vi "Welcome.vi"() -> ()   [LabVIEW 2017]
uses:
  Global/Global 1.vi
  Global/Login Details.vi
  Control/WELCOM SCREEN ENUM.ctl
panel:
  out "Screen Index":i32
  in  "Check 2":bool
  in  "auto":bool
  in  "Test Print":bool
  in  "andon":bool
  in  "MANUAL":bool
  out "error out 2":errorcluster
  in  "error in (no error) 3":errorcluster
  in  "Remove":bool
  in  "Check":bool
  in  "Home":bool
  out "user name":string
  out "STOP":bool
  in  "Tab Control":enum32{"Page 1", "user mangement"}(tab)
  out "error out":errorcluster
  in  "error in (no error)":errorcluster
  in  "LOGIN":bool
  in  "RECIPE":bool
  in  "EXIT":bool
  in  "REPORT":bool
  in  "Hardware Setting":bool
  in  "Shift Setting":bool
  in  "AUTO MODE":bool
  in  "USER MANGMENT":bool
  out "datetime":string
  # "PV Clean Mobility Technologies Traceability System"
  # "USER :"
  # "Powered By - NiVision Automation Systems Pvt. Ltd."
  # "Powered By-Infinity Automation Systems Pvt Ltd. Pune"
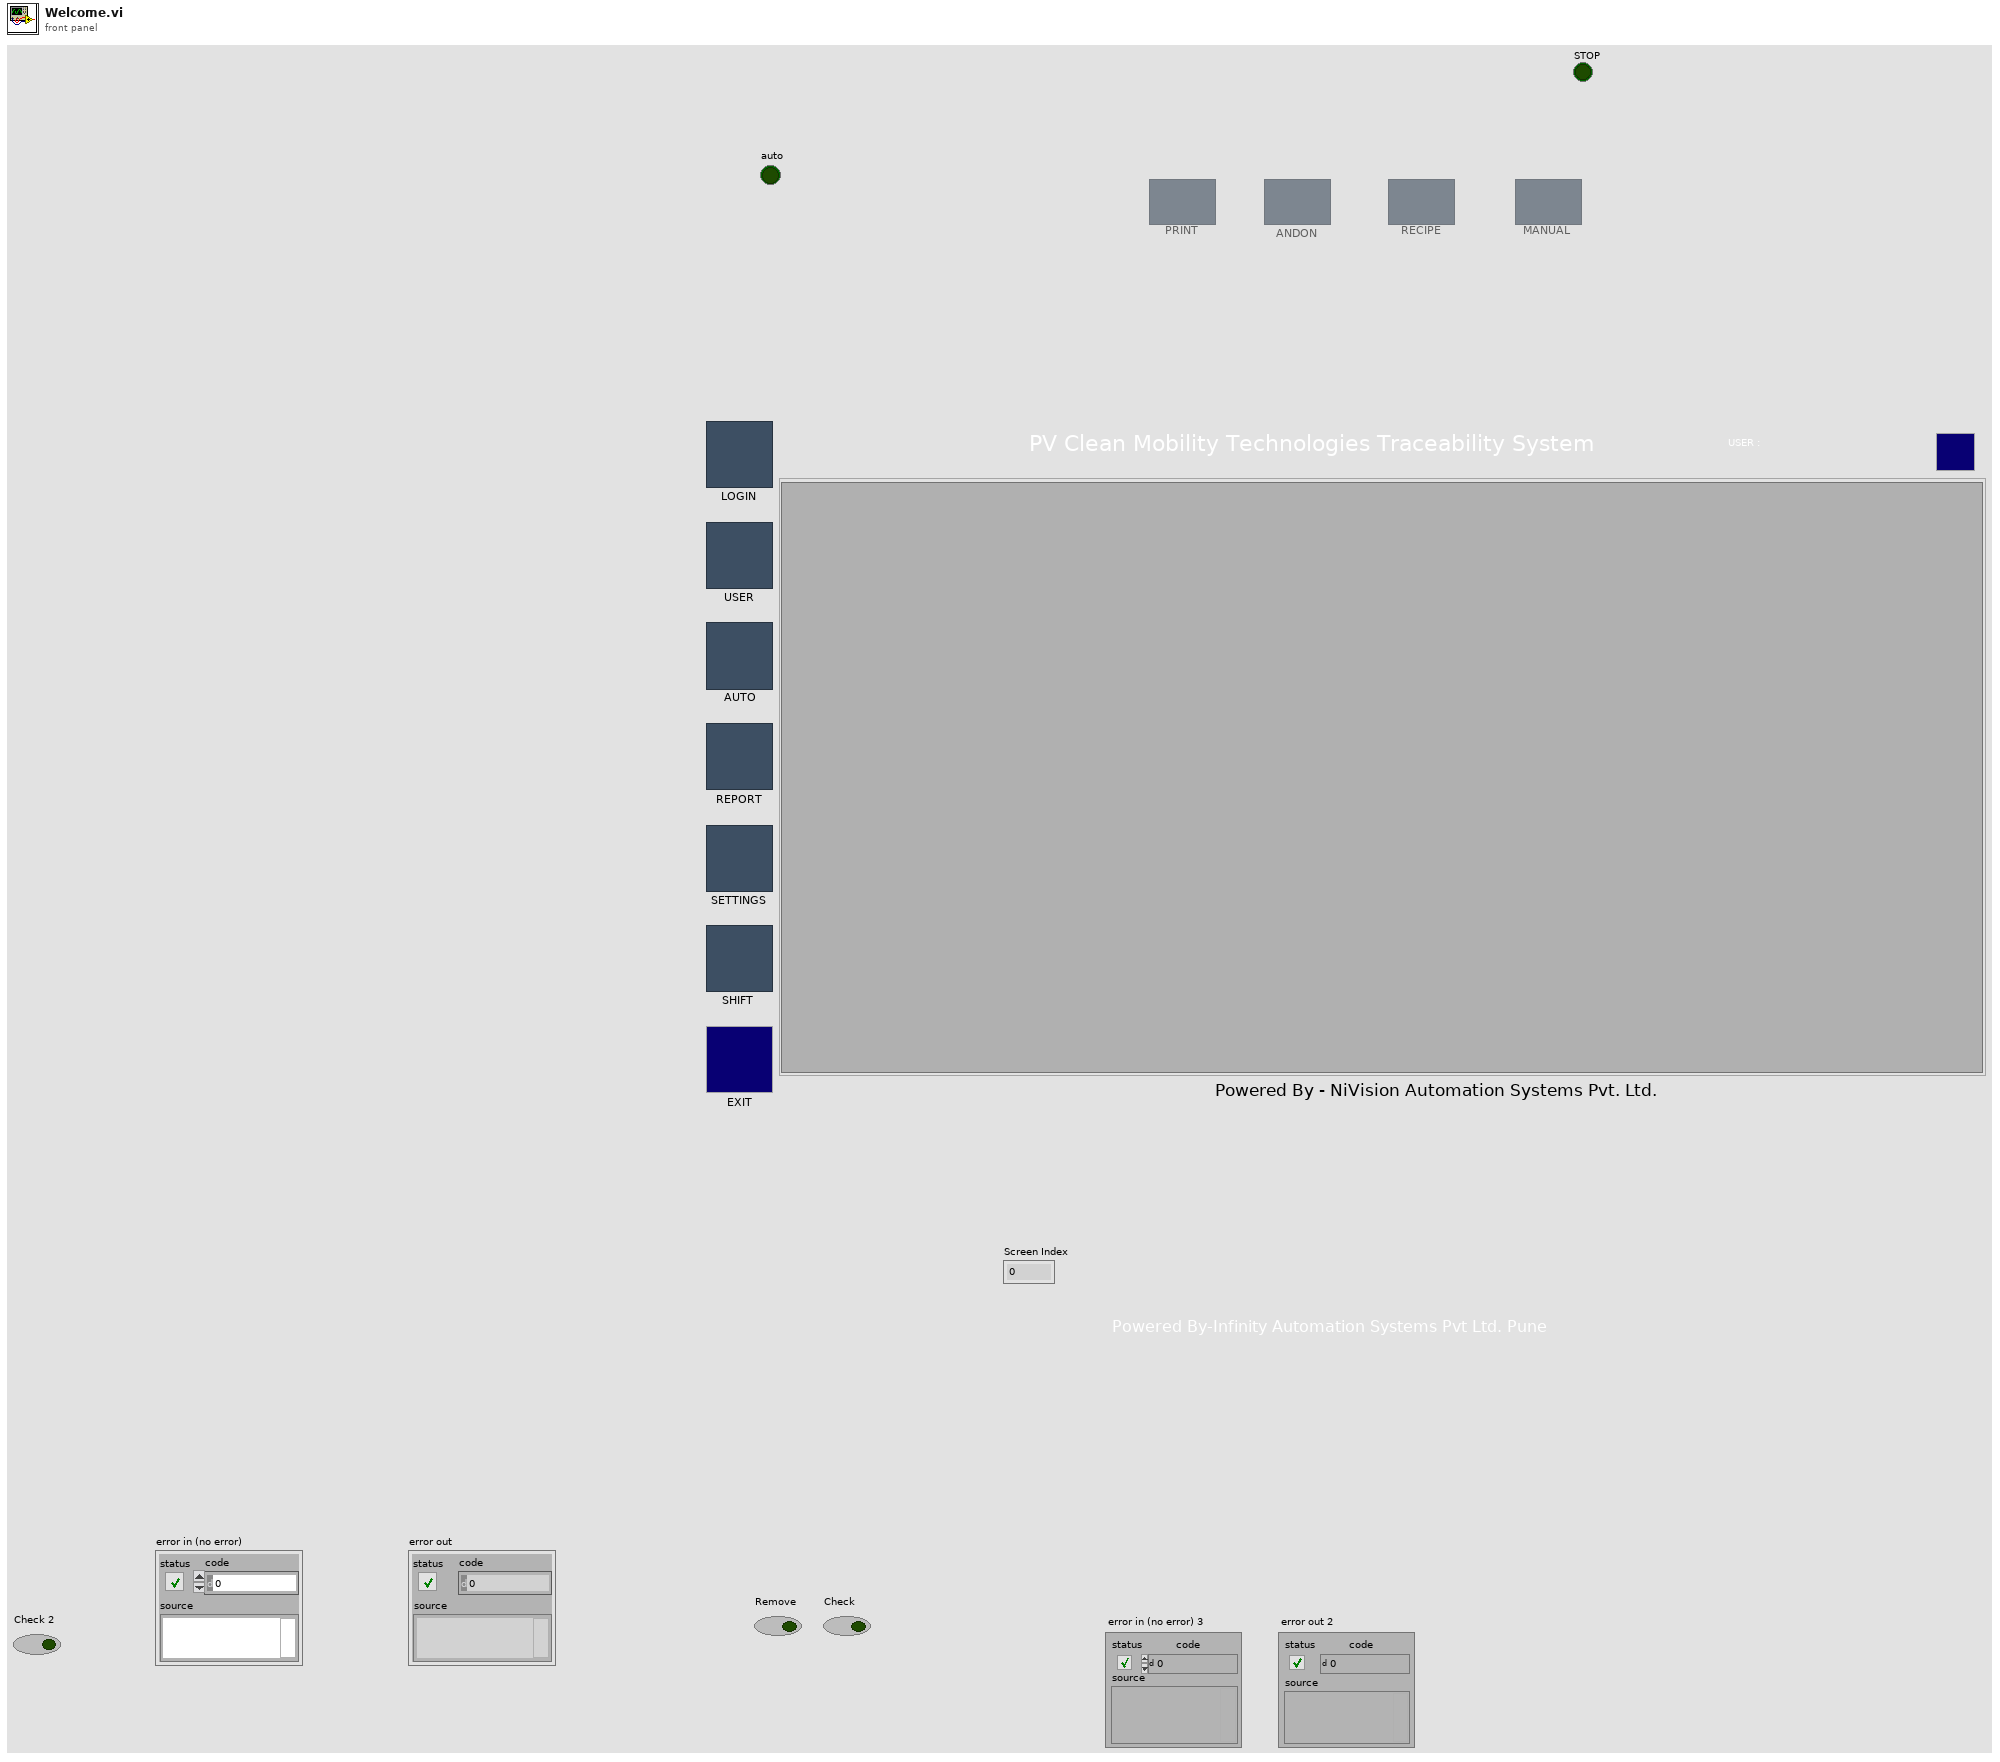
[diagram p1: front panel]
types:
  T1 = typedef "WELCOM SCREEN ENUM.ctl" = enum16{"Initialization", "Wait For Event", "RUN", "LOGIN", "USER MANAGEMENT", "AUTORITY MANAGEMENT", "AUTO MODE", "MANUAL MODE", "BIN MASTER", "CHEMICAL MASTER", "RAW MATERIAL INWARD", "RECIPE INGREDIENT", "REPORT", "SHIFT SETTING", "HARDWARE SETTING", "Check Authority", "TEST PRINT", "EXIT"}
  T2 = cluster{"SCREEN 1":bool, "SCREEN 2":bool, "SCREEN 3":bool, "SCREEN 4":bool, "SCREEN 5":bool, "SCREEN 6":bool, "SCREEN 7":bool, "SCREEN 8":bool, "SCREEN 9":bool, "SCREEN 10":bool, "SCREEN 11":bool, "SCREEN 12":bool, "SCREEN 13":bool, "SCREEN 14":bool, "SCREEN 15":bool, "SCREEN 16":bool, "SCREEN 17":bool, "SCREEN 18":bool, "SCREEN 19":bool, "SCREEN 20":bool}
  T3 = enum8{"Enabled", "Disabled", "Disabled and Grayed Out"}
  T4 = enum32{"Invalid", "Standard", "Closed", "Hidden", "Minimized", "Maximized"}
  T5 = enum32{"Bad", "Idle", "Run top level", "Running"}
  T6 = enum32{"invalid app kind", "Development System", "Run Time System", "Student Edition", "Embedded LabVIEW", "Evaluation", "Custom"}
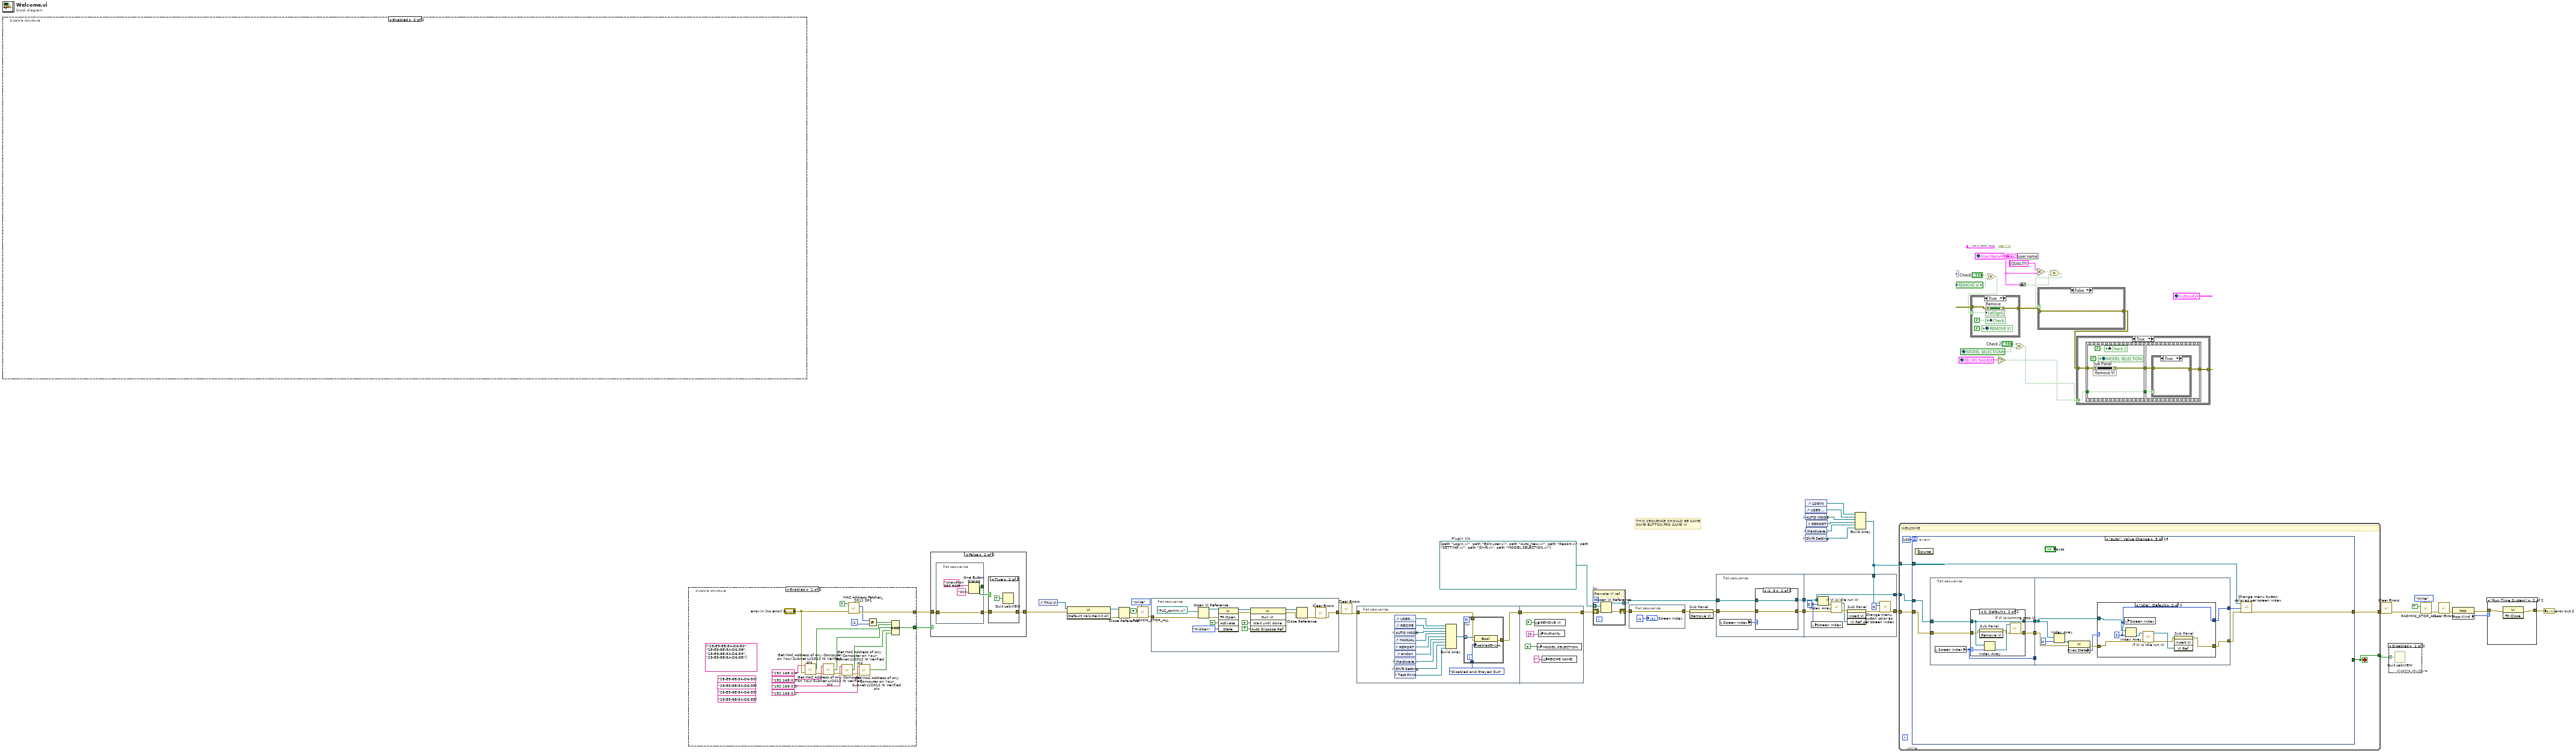
[diagram p0: block diagram]
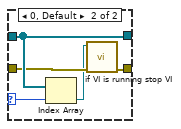
[diagram p2: hidden frame]
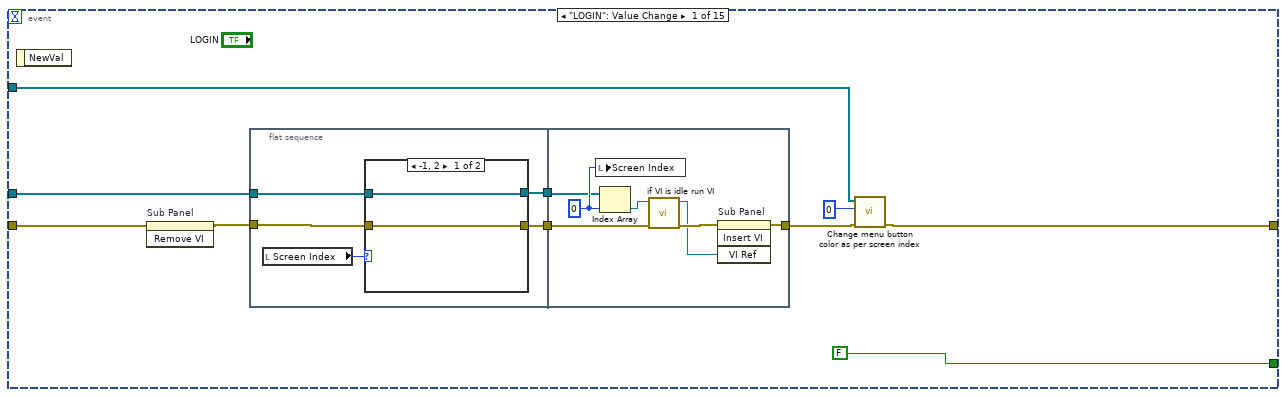
[diagram p5: hidden frame]
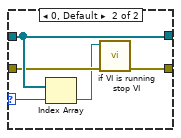
[diagram p6: hidden frame]
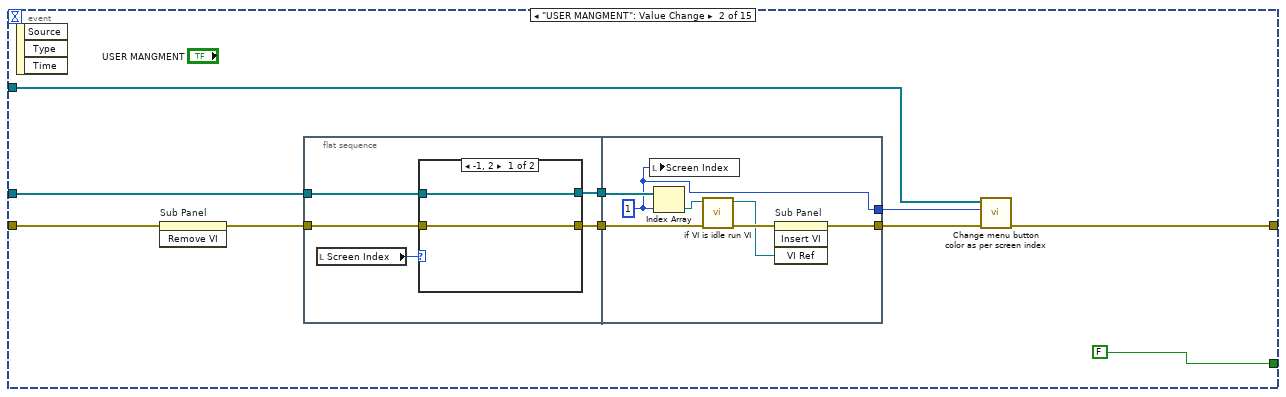
[diagram p7: hidden frame]
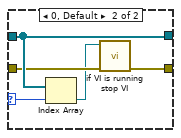
[diagram p8: hidden frame]
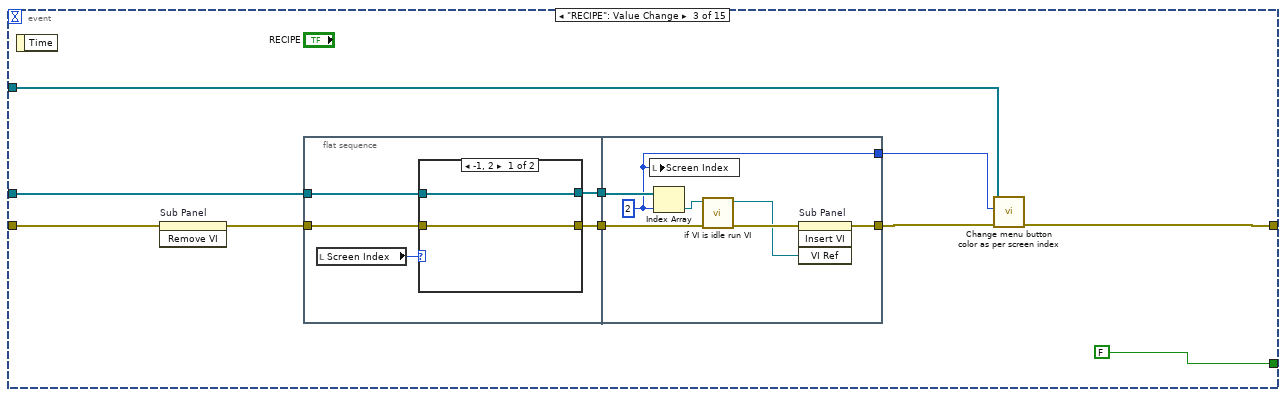
[diagram p9: hidden frame]
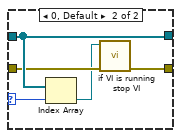
[diagram p10: hidden frame]
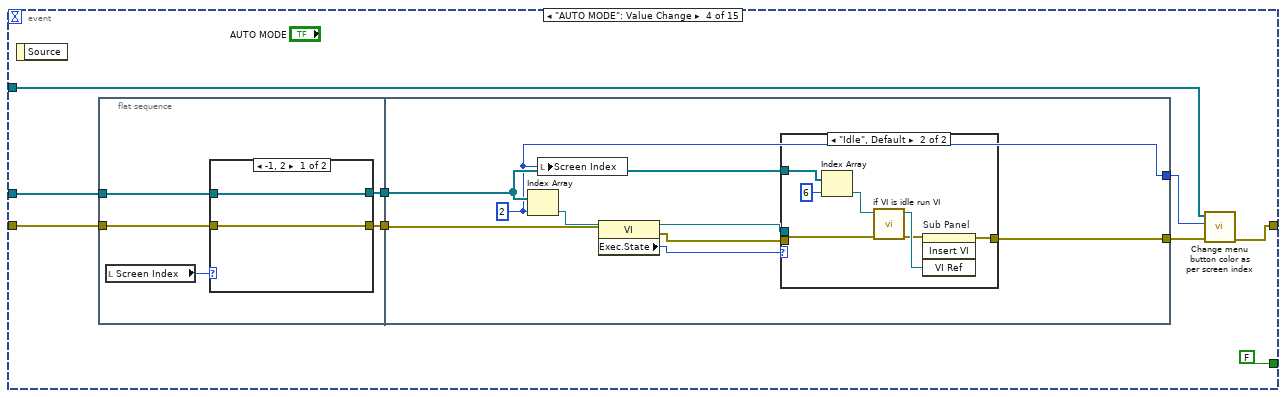
[diagram p11: hidden frame]
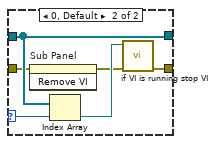
[diagram p12: hidden frame]
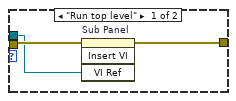
[diagram p13: hidden frame]
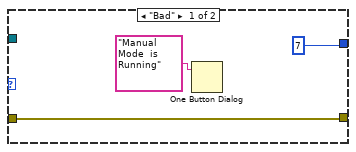
[diagram p15: hidden frame]
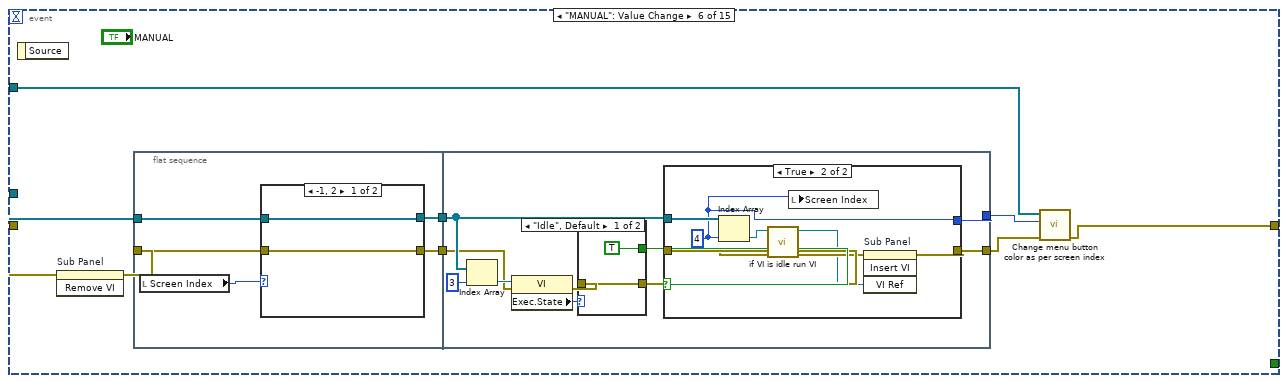
[diagram p16: hidden frame]
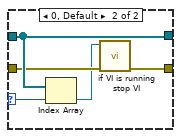
[diagram p17: hidden frame]
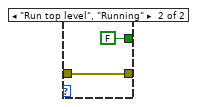
[diagram p18: hidden frame]
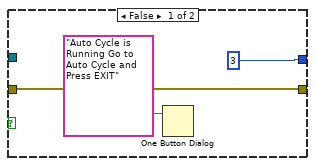
[diagram p19: hidden frame]
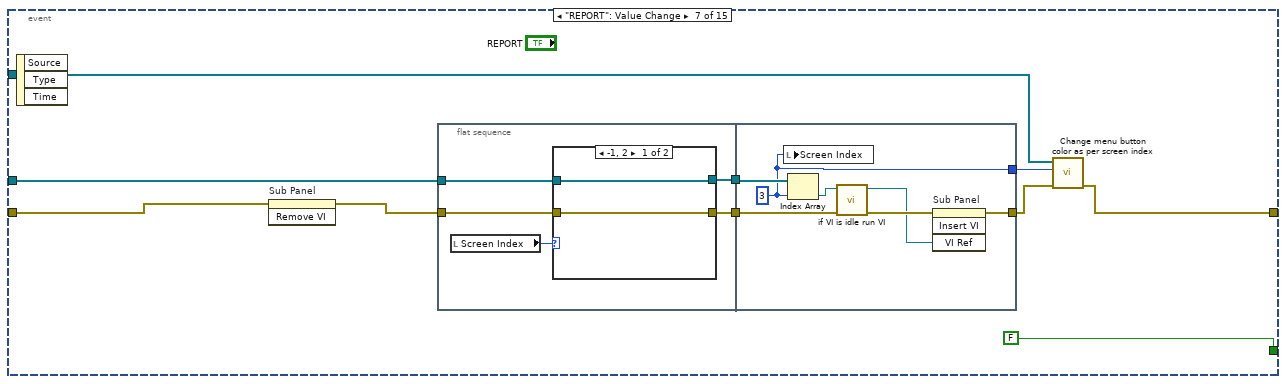
[diagram p20: hidden frame]
diagram:
  w33 = path[] [path "Login.vi", path "Edit user.vi", path "Auto_New.vi", path "Report.vi", path "SETTING.vi", path "Shift.vi", path "MODEL SELECTION.vi"]  # Plugin VIs
  # "THIS SEQUENCE SHOULD BE SAME\nSAME BUTTON FRO SAME VI"
  # "THIS SEQUENCE SHOULD BE SAME\nSAME BUTTON FRO SAME VI"
  n1 = disable-structure shown="Enabled" {
    frame Disabled {
      n2 = flat-sequence {
        tunnel: "error in (no error)" -> [w68]
        tunnel: [w67] -> w43
        frame #0 {
          n3 = invoke class="VI" method="Default Vals.Reinit All"(error in=w68) -> (error out=w67:errorcluster)  [unwired: 2 in, 2 out]
          n4 = global write "Login Details.vi" "Authority"(T2 {"SCREEN 1"=FALSE, "SCREEN 2"=FALSE, "SCREEN 3"=FALSE, "SCREEN 4"=FALSE, "SCREEN 5"=FALSE, "SCREEN 6"=FALSE, "SCREEN 7"=FALSE, "SCREEN 8"=FALSE, "SCREEN 9"=FALSE, "SCREEN 10"=FALSE, "SCREEN 11"=FALSE, "SCREEN 12"=FALSE, "SCREEN 13"=FALSE, "SCREEN 14"=FALSE, "SCREEN 15"=FALSE, "SCREEN 16"=FALSE, "SCREEN 17"=FALSE, "SCREEN 18"=FALSE, "SCREEN 19"=FALSE, "SCREEN 20"=FALSE} ("Authority")) -> ()
        }
      }
      n5 = invoke on="Sub Panel" class="SubPnl" method="Remove VI"(error in=w43) -> (error out=w56:errorcluster)  [unwired: 2 in, 2 out]
      n6 = Open VI Reference(vi path=path "Login.vi", error in (no error)=w56) -> (vi reference=w55:refnum<vi>, error out=w53:errorcluster)  [unwired: 4 in]
      n7 = invoke on="Sub Panel" class="SubPnl" method="Insert VI"(error in=w53, "VI Ref"=w55) -> (error out=w54:errorcluster)  [unwired: 2 in, 3 out]
      n8 = invoke class="VI" method="Run VI"(reference=w55, error in=w54, "Wait until done"=TRUE ("Wait Until Done"), "Auto Dispose Ref"=FALSE ("Auto Dispose Reference")) -> (reference out=w51:refnum<vi>, error out=w52:errorcluster)  [unwired: 1 in, 3 out]
      n9 = Close Reference(reference=w51, error in (no error)=w52) -> (error out=w46:errorcluster)
      n10 = Unbundle By Name(w46) -> ("code"=w50:i32)
      n11 = call <vilib>:"Clear Errors.vi"("error in (no error)"=w46) -> ("error out"=w48:errorcluster)  [unwired: 5 in, 1 out]
      n12 = Not Equal?(x=7, y=w50) -> (x != y?=w49:bool)
      n13 = Select(t=w46, s=w49, f=w48) -> (s? t:f=w47:errorcluster)
      n14 = call <vilib>:"Simple Error Handler.vi"("error in (no error)"=w47) -> ("error out"=w57:errorcluster)  [unwired: 4 in, 4 out]
      n15 = invoke on="Sub Panel" class="SubPnl" method="Remove VI"(error in=w57) -> (error out=w45:errorcluster)  [unwired: 2 in, 2 out]
      n16 = while {
        tunnel: w45 -> [w75]
        shift-right: [w77] -> _
        shift-left: WELCOM_SCREEN_ENUM."Initialization" -> [w71]
        shift-right: [w74] -> _
        shift-left: cluster{"VI Run":string} {"VI Run"=""} -> [w73]
        tunnel: [w76] -> w63
        stop <- w72 stop-if-true
        n17 = case shown="\"AUTORITY MANAGEMENT\"" w71 {
          tunnel: [WELCOM_SCREEN_ENUM."Check Authority" w102 WELCOM_SCREEN_ENUM."Wait For Event" WELCOM_SCREEN_ENUM."Wait For Event" WELCOM_SCREEN_ENUM."RUN" WELCOM_SCREEN_ENUM."RUN" WELCOM_SCREEN_ENUM."RUN" WELCOM_SCREEN_ENUM."RUN" WELCOM_SCREEN_ENUM."RUN" WELCOM_SCREEN_ENUM."RUN" WELCOM_SCREEN_ENUM."RUN" WELCOM_SCREEN_ENUM."RUN" WELCOM_SCREEN_ENUM."RUN" WELCOM_SCREEN_ENUM."RUN" WELCOM_SCREEN_ENUM."RUN" WELCOM_SCREEN_ENUM."RUN" WELCOM_SCREEN_ENUM."RUN" w229] -> w77
          tunnel: [w95 w101 w123 w127 w133 w139 w145 w151 w157 w163 w169 w175 w181 w187 w193 w199 w205 w224] -> w76
          tunnel: w75 -> [w95 w101 w123 w127 w133 w139 w145 w151 w157 w163 w169 w175 w181 w187 w193 w199 w205 w223]
          tunnel: [w93 w99 w122 w126 w131 w137 w142 w146 w155 w161 w167 w170 w177 w185 w188 w194 w203 w222] -> w74
          tunnel: w73 -> [w93 w99 w122 w126 w132 w138 w143 w147 w156 w162 w168 w171 w178 w186 w189 w195 w204 w222]
          tunnel: [FALSE FALSE FALSE TRUE FALSE FALSE FALSE FALSE FALSE FALSE FALSE FALSE FALSE FALSE FALSE FALSE FALSE FALSE] -> w72
          frame "Initialization", Default {
            n18 = control-ref of="USER MANGMENT"() -> (w80:refnum<vi>)
            n19 = control-ref of="RECIPE"() -> (w81:refnum<vi>)
            n20 = control-ref of="AUTO MODE"() -> (w82:refnum<vi>)
            n21 = control-ref of="REPORT"() -> (w88:refnum<vi>)
            n22 = control-ref of="Shift Setting"() -> (w89:refnum<vi>)
            n23 = control-ref of="Hardware Setting"() -> (w90:refnum<vi>)
            n24 = Build Array(w80, w81, w82, w88, w89, w90) -> (w79:refnum<vi>[], w83:refnum<vi>, w84:refnum<vi>, w85:refnum<vi>, w86:refnum<vi>, w87:refnum<vi>, w91:refnum<vi>)
            n25 = for {
              tunnel: w79 -> [w97] mode=indexing
              n26 = property class="Bool"(reference=w97, "DisabledEnum"=T3."Disabled and Grayed Out" ("Disabled")) -> ()  [unwired: 1 in, 2 out]
            }
          }
          frame "Wait For Event" {
            n27 = Search 1D Array(1D array=bool[] [], element=TRUE) -> (index of element=w104:i32)  [unwired: 1 in]
            n28 = case shown="11" w104 {
              tunnel: [WELCOM_SCREEN_ENUM."Wait For Event" WELCOM_SCREEN_ENUM."EXIT" WELCOM_SCREEN_ENUM."LOGIN" WELCOM_SCREEN_ENUM."USER MANAGEMENT" WELCOM_SCREEN_ENUM."AUTORITY MANAGEMENT" WELCOM_SCREEN_ENUM."AUTO MODE" WELCOM_SCREEN_ENUM."MANUAL MODE" WELCOM_SCREEN_ENUM."BIN MASTER" WELCOM_SCREEN_ENUM."CHEMICAL MASTER" WELCOM_SCREEN_ENUM."RAW MATERIAL INWARD" WELCOM_SCREEN_ENUM."REPORT" WELCOM_SCREEN_ENUM."SHIFT SETTING" WELCOM_SCREEN_ENUM."HARDWARE SETTING" WELCOM_SCREEN_ENUM."TEST PRINT" WELCOM_SCREEN_ENUM."RECIPE INGREDIENT"] -> w102
              frame -1, Default {
              }
              frame 0 {
              }
              frame 1 {
              }
              frame 2 {
              }
              frame 3 {
              }
              frame 4 {
              }
              frame 5 {
              }
              frame 6 {
              }
              frame 7 {
              }
              frame 8 {
              }
              frame 9 {
              }
              frame 10 {
              }
              frame 11 {
              }
              frame 12 {
              }
              frame 13 {
              }
            }
          }
          frame "Check Authority" {
          }
          frame "EXIT" {
          }
          frame "LOGIN" {
            w130 = "Login.vi"  # VI Run
            n29 = Bundle By Name(cluster=w132, "VI Run"=w130) -> (w131:cluster{"VI Run":string})
          }
          frame "USER MANAGEMENT" {
            w136 = "User Management.vi"  # VI Run
            n30 = Bundle By Name(cluster=w138, "VI Run"=w136) -> (w137:cluster{"VI Run":string})
          }
          frame "AUTORITY MANAGEMENT" {
            w141 = "Authority Management.vi"  # VI Run
            n31 = Bundle By Name(cluster=w143, "VI Run"=w141) -> (w142:cluster{"VI Run":string})
          }
          frame "AUTO MODE" {
            w148 = "AUTO MODE.vi"  # VI Run
            n32 = Bundle By Name(cluster=w147, "VI Run"=w148) -> (w146:cluster{"VI Run":string})
          }
          frame "MANUAL MODE" {
            w154 = "Manual Mode.vi"  # VI Run
            n33 = Bundle By Name(cluster=w156, "VI Run"=w154) -> (w155:cluster{"VI Run":string})
          }
          frame "BIN MASTER" {
            w160 = "Bin Master.vi"  # VI Run
            n34 = Bundle By Name(cluster=w162, "VI Run"=w160) -> (w161:cluster{"VI Run":string})
          }
          frame "CHEMICAL MASTER" {
            w166 = "Chemical Master.vi"  # VI Run
            n35 = Bundle By Name(cluster=w168, "VI Run"=w166) -> (w167:cluster{"VI Run":string})
          }
          frame "RAW MATERIAL INWARD" {
            w172 = "raw material inward.vi"  # VI Run
            n36 = Bundle By Name(cluster=w171, "VI Run"=w172) -> (w170:cluster{"VI Run":string})
          }
          frame "RECIPE INGREDIENT" {
            w179 = "Recipe_Ingredients.vi"  # VI Run
            n37 = Bundle By Name(cluster=w178, "VI Run"=w179) -> (w177:cluster{"VI Run":string})
          }
          frame "REPORT" {
            w184 = "Report.vi"  # VI Run
            n38 = Bundle By Name(cluster=w186, "VI Run"=w184) -> (w185:cluster{"VI Run":string})
          }
          frame "SHIFT SETTING" {
            w190 = "shift setting.vi"  # VI Run
            n39 = Bundle By Name(cluster=w189, "VI Run"=w190) -> (w188:cluster{"VI Run":string})
          }
          frame "HARDWARE SETTING" {
            w196 = "Hardware Setting.vi"  # VI Run
            n40 = Bundle By Name(cluster=w195, "VI Run"=w196) -> (w194:cluster{"VI Run":string})
          }
          frame "TEST PRINT" {
            w202 = "Test Print.vi"  # VI Run
            n41 = Bundle By Name(cluster=w204, "VI Run"=w202) -> (w203:cluster{"VI Run":string})
          }
          frame "RUN" {
            w230 = "Login.vi"  # x
            n42 = Unbundle By Name(w222) -> ("VI Run"=w231:string)
            n43 = invoke on="Sub Panel" class="SubPnl" method="Remove VI"(error in=w223) -> (error out=w212:errorcluster)  [unwired: 2 in, 2 out]
            n44 = Equal?(x=w230, y=w231) -> (x = y?=w228:bool)
            n45 = String To Path(string=w231) -> (path=w207:path)
            n46 = Open VI Reference(vi path=w207, error in (no error)=w212) -> (vi reference=w213:refnum<vi>, error out=w215:errorcluster)  [unwired: 4 in]
            n47 = invoke on="Sub Panel" class="SubPnl" method="Insert VI"(error in=w215, "VI Ref"=w213) -> (error out=w214:errorcluster)  [unwired: 2 in, 3 out]
            n48 = invoke class="VI" method="Run VI"(reference=w213, error in=w214, "Wait until done"=TRUE ("Wait Until Done"), "Auto Dispose Ref"=FALSE ("Auto Dispose Reference")) -> (reference out=w217:refnum<vi>, error out=w216:errorcluster)  [unwired: 1 in, 3 out]
            n49 = Close Reference(reference=w217, error in (no error)=w216) -> (error out=w206:errorcluster)
            n50 = Unbundle By Name(w206) -> ("code"=w218:i32)
            n51 = call <vilib>:"Clear Errors.vi"("error in (no error)"=w206) -> ("error out"=w220:errorcluster)  [unwired: 5 in, 1 out]
            n52 = Not Equal?(x=7, y=w218) -> (x != y?=w219:bool)
            n53 = Select(t=WELCOM_SCREEN_ENUM."Check Authority", s=w228, f=WELCOM_SCREEN_ENUM."Wait For Event") -> (s? t:f=w229:T1)
            n54 = Select(t=w206, s=w219, f=w220) -> (s? t:f=w221:errorcluster)
            n55 = call <vilib>:"Simple Error Handler.vi"("error in (no error)"=w221) -> ("error out"=w211:errorcluster)  [unwired: 4 in, 4 out]
            n56 = invoke on="Sub Panel" class="SubPnl" method="Remove VI"(error in=w211) -> (error out=w224:errorcluster)  [unwired: 2 in, 2 out]
          }
        }
        "STOP" <- w72
        n57 = Wait (ms)(milliseconds to wait=u32 100) -> ()  [unwired: 1 out]
      }
      n58 = while {
        tunnel: w43 -> [w65]
        tunnel: [w65] -> w41
        stop <- w66 stop-if-true
        n59 = local read "STOP"() -> (w66:bool)
      }
      n60 = Merge Errors(w41, w63) -> (→"error out":errorcluster)
      n61 = disable-structure shown="Enabled" {
        disable-tunnel: w63 -> [w70 _]
        frame Enabled {
          n62 = invoke class="VI" method="FP.Close"(error in=w70) -> ()  [unwired: 2 in, 3 out]
        }
        frame Disabled {
        }
      }
    }
    frame Enabled {
    }
  }
  n63 = disable-structure shown="Enabled" {
    disable-tunnel: [w248 _] -> w4
    disable-tunnel: [w236 TRUE] -> w2
    frame Enabled {
      (unwired) string[] ["28-E9-8E-5A-D6-50", "28-E9-8E-5A-D6-3B", "28-E9-8E-5A-D6-59", "28-E9-8E-5A-D6-5E"]
      (unwired) "28-E9-8E-5A-D6-5E" ("IP Address")
      (unwired) "28-E9-8E-5A-D6-59" ("IP Address")
      (unwired) "28-E9-8E-5A-D6-3B" ("IP Address")
      (unwired) "28-E9-8E-5A-D6-50" ("IP Address")
      n64 = call "Get MAC Address of Any Computer on Your Subnet LV2012 NI Verified plc.vi"("error constant"="error in (no error) 3", "IP Address"="192.168.0.4") -> ("error out"=w244:errorcluster, "x .and. y?"=w235:bool)  [unwired: 1 in, 1 out]
      n65 = call "Get MAC Address of Any Computer on Your Subnet LV2012 NI Verified plc.vi"("error constant"=w244, "IP Address"="192.168.0.3") -> ("error out"=w242:errorcluster, "x .and. y?"=w234:bool)  [unwired: 1 in, 1 out]
      n66 = call "Get MAC Address of Any Computer on Your Subnet LV2012 NI Verified plc.vi"("error constant"=w242, "IP Address"="192.168.0.2") -> ("error out"=w243:errorcluster, "x .and. y?"=w233:bool)  [unwired: 1 in, 1 out]
      n67 = call "MAC Address Fetcher_2011 SP1.vi"("error in (no error)"="error in (no error) 3", "Search all adapters?"=TRUE) -> ("error out"=w248:errorcluster, "index of element"=w239:i32)  [unwired: 6 in, 2 out]
      n68 = call "Get MAC Address of Any Computer on Your Subnet LV2012 NI Verified plc.vi"("error constant"=w243, "IP Address"="192.168.0.1") -> ("x .and. y?"=w232:bool)  [unwired: 1 in, 2 out]
      n69 = Not Equal?(x=w239, y=-1) -> (x != y?=w237:bool)
      n70 = Compound Arithmetic op=AND(w237, w235, w234, w233, w232) -> (w236:bool)
    }
    frame Disabled {
    }
  }
  n71 = case shown="False" w2 {
    tunnel: w4 -> [w252 w262]
    tunnel: [w251 w262] -> w3
    frame False {
      n72 = flat-sequence {
        tunnel: [w257] -> w254
        tunnel: [w256] -> w253
        tunnel: w252 -> [w256]
        frame #0 {
          n73 = One Button Dialog(message="Unauthorised access to this system\nPlease contact to NIVision Automation Systems Pvt Ltd", button name ("OK")="OK") -> (true=w257:bool)
        }
      }
      n74 = case shown="True" w254 {
        tunnel: w253 -> [w259 w260]
        tunnel: [w259 w260] -> w251
        frame False {
        }
        frame True {
          n75 = Quit LabVIEW(quit? (T)=TRUE) -> ()
        }
      }
    }
    frame True {
    }
  }
  n76 = control-ref of="This VI"() -> (w40:refnum<vi>)
  n77 = invoke class="VI" method="Default Vals.Reinit All"(reference=w40, error in=w3) -> (reference out=w38:refnum<vi>, error out=w39:errorcluster)  [unwired: 1 in, 1 out]
  n78 = Close Reference(reference=w38, error in (no error)=w39) -> (error out=w6:errorcluster)
  n79 = call "PADMINI_STOP_ALL.vi"("Enum"=enum16{"Read", "Write"}."Write", "error in (no error)"=w6, "Boolean"=FALSE) -> ("error out"=w5:errorcluster)  [unwired: 7 in, 1 out]
  n80 = flat-sequence {
    tunnel: w5 -> [w276]
    tunnel: [w274] -> w21
    frame #0 {
      n81 = Open VI Reference(vi path=path "PLC_comm.vi", error in (no error)=w276) -> (vi reference=w267:refnum<vi>, error out=w268:errorcluster)  [unwired: 4 in]
      n82 = invoke class="VI" method="FP.Open"(reference=w267, error in=w268, "Activate"=TRUE ("Activate?"), "State"=T4."Hidden") -> (reference out=w270:refnum<vi>, error out=w269:errorcluster)  [unwired: 1 in, 3 out]
      n83 = invoke class="VI" method="Run VI"(reference=w270, error in=w269, "Wait until done"=FALSE ("Wait Until Done"), "Auto Dispose Ref"=TRUE ("Auto Dispose Reference")) -> (reference out=w265:refnum<vi>, error out=w264:errorcluster)  [unwired: 1 in, 3 out]
      n84 = Close Reference(reference=w265, error in (no error)=w264) -> (error out=w275:errorcluster)
      n85 = call <vilib>:"Clear Errors.vi"("error in (no error)"=w275) -> ("error out"=w274:errorcluster)  [unwired: 5 in, 1 out]
    }
  }
  n86 = call <vilib>:"Clear Errors.vi"("error in (no error)"=w21) -> ("error out"=w20:errorcluster)  [unwired: 5 in, 1 out]
  n87 = flat-sequence {
    tunnel: w20 -> [w278]
    tunnel: [w277] -> w13
    tunnel: [w298] -> w23
    tunnel: w13 -> [w298]
    frame #0 {
      n88 = control-ref of="Shift Setting"() -> (w282:refnum<vi>)
      n89 = control-ref of="Test Print"() -> (w281:refnum<vi>)
      n90 = control-ref of="USER MANGMENT"() -> (w289:refnum<vi>)
      n91 = control-ref of="RECIPE"() -> (w288:refnum<vi>)
      n92 = control-ref of="AUTO MODE"() -> (w287:refnum<vi>)
      n93 = control-ref of="MANUAL"() -> (w286:refnum<vi>)
      n94 = control-ref of="REPORT"() -> (w285:refnum<vi>)
      n95 = control-ref of="andon"() -> (w284:refnum<vi>)
      n96 = control-ref of="Hardware Setting"() -> (w283:refnum<vi>)
      n97 = Build Array(w289, w288, w287, w286, w285, w284, w283, w282, w281) -> (w280:refnum<vi>[])
      n98 = for {
        tunnel: w280 -> [w293] mode=indexing
        tunnel: w278 -> [w292]
        tunnel: T3."Disabled and Grayed Out" ("Disabled") -> [w291]
        tunnel: [w290] -> w277
        n99 = property class="Bool"(reference=w293, error in=w292, "DisabledEnum"=w291) -> (error out=w290:errorcluster)  [unwired: 1 out]
      }
    }
    frame #1 {
      n100 = global write "Global 1.vi" "REMOVE VI"(FALSE ("REMOVE VI")) -> ()
      n101 = global write "Global 1.vi" "MODEL SELECTION"(FALSE ("REMOVE VI")) -> ()
      n102 = global write "Login Details.vi" "Authority"(T2 {"SCREEN 1"=FALSE, "SCREEN 2"=FALSE, "SCREEN 3"=FALSE, "SCREEN 4"=FALSE, "SCREEN 5"=FALSE, "SCREEN 6"=FALSE, "SCREEN 7"=FALSE, "SCREEN 8"=FALSE, "SCREEN 9"=FALSE, "SCREEN 10"=FALSE, "SCREEN 11"=FALSE, "SCREEN 12"=FALSE, "SCREEN 13"=FALSE, "SCREEN 14"=FALSE, "SCREEN 15"=FALSE, "SCREEN 16"=FALSE, "SCREEN 17"=FALSE, "SCREEN 18"=FALSE, "SCREEN 19"=FALSE, "SCREEN 20"=FALSE} ("Authority")) -> ()
      n103 = global write "Global 1.vi" "RECIPE NAME"("" ("RECIPE NAME")) -> ()
    }
  }
  n104 = for {
    tunnel: w33 -> [w300] mode=indexing
    tunnel: [w301] -> w26 mode=indexing
    shift-right: [w302] -> w32
    shift-left: w23 -> [w299]
    # "Genrate VI ref."
    n105 = Open VI Reference(vi path=w300, error in (no error)=w299) -> (vi reference=w301:refnum<vi>, error out=w302:errorcluster)  [unwired: 4 in]
  }
  n106 = flat-sequence {
    tunnel: w32 -> [w304]
    tunnel: [w304] -> w28
    frame #0 {
      "Screen Index" <- -1 ("Screen Index")
    }
  }
  n107 = invoke on="Sub Panel" class="SubPnl" method="Remove VI"(error in=w28) -> (error out=w29:errorcluster)  [unwired: 2 in, 2 out]
  n108 = flat-sequence {
    tunnel: w26 -> [w307]
    tunnel: [w309] -> w31
    tunnel: [w306] -> w30
    tunnel: w29 -> [w305]
    tunnel: w31 -> [w325]
    tunnel: w30 -> [w321]
    tunnel: [w318] -> w27
    tunnel: [w321] -> w25
    tunnel: w24 -> [w317]
    frame #0 {
      n109 = local read "Screen Index"() -> (w308:i32)
      n110 = case shown="-1, 3" w308 {
        selector: w308 -> [_ w316]
        tunnel: w305 -> [w311 w314]
        tunnel: [w311 w313] -> w309
        tunnel: w307 -> [w310 w315]
        tunnel: [w310 w315] -> w306
        frame -1, 3 {
        }
        frame 0, Default {
          n111 = Index Array(array=w315, index=w316) -> (element=w312:refnum<vi>)
          n112 = call "if VI is running stop VI.vi"("error in (no error)"=w314, "VI in"=w312) -> ("error out"=w313:errorcluster)  [unwired: 8 in, 1 out]
        }
      }
    }
    frame #1 {
      w326 = 0 ("index")
      n113 = local write "Screen Index"(w326) -> ()
      n114 = Index Array(array=w321, index=w326) -> (element=w324:refnum<vi>)
      n115 = call "if VI is idle run VI.vi"("error in (no error)"=w325, "VI in"=w324) -> ("error out"=w323:errorcluster, "VI out"=w322:refnum<vi>)  [unwired: 8 in]
      n116 = invoke on="Sub Panel" class="SubPnl" method="Insert VI"(error in=w323, "VI Ref"=w322) -> (error out=w319:errorcluster)  [unwired: 2 in, 3 out]
      n117 = call "Change menu button color as per screen index.vi"("error in (no error)"=w319, "Screen Index"=0, "Array"=w317) -> ("error out"=w318:errorcluster)  [unwired: 8 in]
    }
  }
  n118 = control-ref of="LOGIN"() -> (w19:refnum<vi>)
  n119 = control-ref of="USER MANGMENT"() -> (w18:refnum<vi>)
  n120 = control-ref of="AUTO MODE"() -> (w17:refnum<vi>)
  n121 = control-ref of="Shift Setting"() -> (w14:refnum<vi>)
  n122 = control-ref of="Hardware Setting"() -> (w15:refnum<vi>)
  n123 = control-ref of="REPORT"() -> (w16:refnum<vi>)
  n124 = Build Array(w19, w18, w17, w16, w15, w14) -> (w24:refnum<vi>[])
  n125 = while {
    tunnel: w27 -> [w329]
    tunnel: [w331] -> w22
    tunnel: w25 -> [w328]
    tunnel: w24 -> [w330]
    tunnel: [w327] -> w1
    stop <- w327 stop-if-true
    # "WELCOME"
    n126 = event shown="[4] \"auto\": Value Change" {
      selector: _ -> [_ _ _ _ _ _ _ _ _ _ _ _ _ _ _]
      dyn-events: _ -> [_ _ _ _ _ _ _ _ _ _ _ _ _ _ _]
      timeout: 100 -> [_ _ _ _ _ _ _ _ _ _ _ _ _ _ _]
      tunnel: [FALSE FALSE FALSE FALSE _ _ FALSE FALSE FALSE FALSE FALSE FALSE w697 FALSE FALSE] -> w327
      tunnel: [w335 w366 w395 w427 w460 w500 w549 w578 w607 w636 w665 w692 w696 w737 w740] -> w331
      tunnel: w328 -> [w341 w370 w399 w423 w464 w503 w553 w582 w611 w640 w669 _ w698 _ _]
      tunnel: w330 -> [w334 w364 w392 w426 w463 w501 w547 w575 w604 w634 w662 w691 w701 w735 _]
      tunnel: w329 -> [w333 w362 w391 w422 w465 w502 w545 w574 w603 w632 w661 w690 w705 w734 w752]
      event "LOGIN": Value Change {
        n127 = event-data() -> ()  [unwired: 1 in, 1 out]
        n128 = invoke on="Sub Panel" class="SubPnl" method="Remove VI"(error in=w333) -> (error out=w338:errorcluster)  [unwired: 2 in, 2 out]
        n129 = flat-sequence {
          tunnel: w341 -> [w345]
          tunnel: [w347] -> w340
          tunnel: [w344] -> w339
          tunnel: w338 -> [w343]
          tunnel: w340 -> [w359]
          tunnel: w339 -> [w360]
          tunnel: [w355] -> w336
          frame #0 {
            n130 = local read "Screen Index"() -> (w346:i32)
            n131 = case shown="-1, 2" w346 {
              selector: w346 -> [_ w354]
              tunnel: w343 -> [w349 w352]
              tunnel: [w349 w351] -> w347
              tunnel: w345 -> [w348 w353]
              tunnel: [w348 w353] -> w344
              frame -1, 2 {
              }
              frame 0, Default {
                n132 = Index Array(array=w353, index=w354) -> (element=w350:refnum<vi>)
                n133 = call "if VI is running stop VI.vi"("error in (no error)"=w352, "VI in"=w350) -> ("error out"=w351:errorcluster)  [unwired: 8 in, 1 out]
              }
            }
          }
          frame #1 {
            w361 = 0 ("index")
            n134 = local write "Screen Index"(w361) -> ()
            n135 = Index Array(array=w360, index=w361) -> (element=w358:refnum<vi>)
            n136 = call "if VI is idle run VI.vi"("error in (no error)"=w359, "VI in"=w358) -> ("error out"=w357:errorcluster, "VI out"=w356:refnum<vi>)  [unwired: 8 in]
            n137 = invoke on="Sub Panel" class="SubPnl" method="Insert VI"(error in=w357, "VI Ref"=w356) -> (error out=w355:errorcluster)  [unwired: 2 in, 3 out]
          }
        }
        n138 = call "Change menu button color as per screen index.vi"("error in (no error)"=w336, "Screen Index"=0, "Array"=w334) -> ("error out"=w335:errorcluster)  [unwired: 8 in]
      }
      event "USER MANGMENT": Value Change {
        n139 = event-data() -> ()  [unwired: 1 in, 3 out]
        n140 = invoke on="Sub Panel" class="SubPnl" method="Remove VI"(error in=w362) -> (error out=w367:errorcluster)  [unwired: 2 in, 2 out]
        n141 = flat-sequence {
          tunnel: w367 -> [w376]
          tunnel: w370 -> [w373]
          tunnel: [w375] -> w369
          tunnel: [w372] -> w368
          tunnel: [w389] -> w365
          tunnel: w369 -> [w388]
          tunnel: w368 -> [w390]
          tunnel: [w384] -> w363
          frame #0 {
            n142 = local read "Screen Index"() -> (w374:i32)
            n143 = case shown="-1, 2" w374 {
              selector: w374 -> [_ w383]
              tunnel: w376 -> [w378 w381]
              tunnel: [w378 w380] -> w375
              tunnel: w373 -> [w377 w382]
              tunnel: [w377 w382] -> w372
              frame -1, 2 {
              }
              frame 0, Default {
                n144 = Index Array(array=w382, index=w383) -> (element=w379:refnum<vi>)
                n145 = call "if VI is running stop VI.vi"("error in (no error)"=w381, "VI in"=w379) -> ("error out"=w380:errorcluster)  [unwired: 8 in, 1 out]
              }
            }
          }
          frame #1 {
            w384 = 1 ("index")
            n146 = local write "Screen Index"(w384) -> ()
            n147 = Index Array(array=w390, index=w384) -> (element=w386:refnum<vi>)
            n148 = call "if VI is idle run VI.vi"("error in (no error)"=w388, "VI in"=w386) -> ("error out"=w387:errorcluster, "VI out"=w385:refnum<vi>)  [unwired: 8 in]
            n149 = invoke on="Sub Panel" class="SubPnl" method="Insert VI"(error in=w387, "VI Ref"=w385) -> (error out=w389:errorcluster)  [unwired: 2 in, 3 out]
          }
        }
        n150 = call "Change menu button color as per screen index.vi"("error in (no error)"=w365, "Screen Index"=w363, "Array"=w364) -> ("error out"=w366:errorcluster)  [unwired: 8 in]
      }
      event "RECIPE": Value Change {
        n151 = event-data() -> ()  [unwired: 1 in, 1 out]
        n152 = invoke on="Sub Panel" class="SubPnl" method="Remove VI"(error in=w391) -> (error out=w396:errorcluster)  [unwired: 2 in, 2 out]
        n153 = flat-sequence {
          tunnel: w396 -> [w405]
          tunnel: w399 -> [w402]
          tunnel: [w404] -> w398
          tunnel: [w401] -> w397
          tunnel: [w418] -> w394
          tunnel: w398 -> [w417]
          tunnel: w397 -> [w419]
          tunnel: [w413] -> w393
          frame #0 {
            n154 = local read "Screen Index"() -> (w403:i32)
            n155 = case shown="-1, 2" w403 {
              selector: w403 -> [_ w412]
              tunnel: w405 -> [w407 w410]
              tunnel: [w407 w409] -> w404
              tunnel: w402 -> [w406 w411]
              tunnel: [w406 w411] -> w401
              frame -1, 2 {
              }
              frame 0, Default {
                n156 = Index Array(array=w411, index=w412) -> (element=w408:refnum<vi>)
                n157 = call "if VI is running stop VI.vi"("error in (no error)"=w410, "VI in"=w408) -> ("error out"=w409:errorcluster)  [unwired: 8 in, 1 out]
              }
            }
          }
          frame #1 {
            w413 = 2 ("index")
            n158 = local write "Screen Index"(w413) -> ()
            n159 = Index Array(array=w419, index=w413) -> (element=w414:refnum<vi>)
            n160 = call "if VI is idle run VI.vi"("error in (no error)"=w417, "VI in"=w414) -> ("error out"=w416:errorcluster, "VI out"=w415:refnum<vi>)  [unwired: 8 in]
            n161 = invoke on="Sub Panel" class="SubPnl" method="Insert VI"(error in=w416, "VI Ref"=w415) -> (error out=w418:errorcluster)  [unwired: 2 in, 3 out]
          }
        }
        n162 = call "Change menu button color as per screen index.vi"("error in (no error)"=w394, "Screen Index"=w393, "Array"=w392) -> ("error out"=w395:errorcluster)  [unwired: 8 in]
      }
      event "AUTO MODE": Value Change {
        n163 = event-data() -> ()  [unwired: 1 in, 1 out]
        n164 = flat-sequence {
          tunnel: w422 -> [w433]
          tunnel: w423 -> [w431]
          tunnel: [w432] -> w425
          tunnel: [w430] -> w424
          tunnel: [w446] -> w420
          tunnel: w425 -> [w449]
          tunnel: w424 -> [w448]
          tunnel: [w447] -> w421
          frame #0 {
            n165 = local read "Screen Index"() -> (w429:i32)
            n166 = case shown="-1, 2" w429 {
              selector: w429 -> [_ w441]
              tunnel: w433 -> [w435 w437]
              tunnel: [w435 w439] -> w432
              tunnel: w431 -> [w434 w440]
              tunnel: [w434 w440] -> w430
              frame -1, 2 {
              }
              frame 0, Default {
                n167 = invoke on="Sub Panel" class="SubPnl" method="Remove VI"(error in=w437) -> (error out=w436:errorcluster)  [unwired: 2 in, 2 out]
                n168 = Index Array(array=w440, index=w441) -> (element=w438:refnum<vi>)
                n169 = call "if VI is running stop VI.vi"("error in (no error)"=w436, "VI in"=w438) -> ("error out"=w439:errorcluster)  [unwired: 8 in, 1 out]
              }
            }
          }
          frame #1 {
            w447 = 2 ("index")
            n170 = Index Array(array=w448, index=w447) -> (element=w442:refnum<vi>)
            n171 = local write "Screen Index"(w447) -> ()
            n172 = property class="VI"(reference=w442, error in=w449) -> (reference out=w443:refnum<vi>, error out=w444:errorcluster, "Exec.State"=w445:T5)
            n173 = case shown="\"Idle\", Default" w445 {
              tunnel: [w452 w457] -> w446
              tunnel: w444 -> [w451 w458]
              tunnel: w443 -> [w450 _]
              tunnel: w448 -> [_ w456]
              frame "Run top level" {
                n174 = invoke on="Sub Panel" class="SubPnl" method="Insert VI"(error in=w451, "VI Ref"=w450) -> (error out=w452:errorcluster)  [unwired: 2 in, 3 out]
              }
              frame "Idle", Default {
                n175 = Index Array(array=w456, index=6) -> (element=w455:refnum<vi>)
                n176 = call "if VI is idle run VI.vi"("error in (no error)"=w458, "VI in"=w455) -> ("error out"=w453:errorcluster, "VI out"=w459:refnum<vi>)  [unwired: 8 in]
                n177 = invoke on="Sub Panel" class="SubPnl" method="Insert VI"(error in=w453, "VI Ref"=w459) -> (error out=w457:errorcluster)  [unwired: 2 in, 3 out]
              }
            }
          }
        }
        n178 = call "Change menu button color as per screen index.vi"("error in (no error)"=w420, "Screen Index"=w421, "Array"=w426) -> ("error out"=w427:errorcluster)  [unwired: 8 in]
      }
      event "auto": Value Change {
        n179 = event-data() -> ()  [unwired: 1 in, 1 out]
        n180 = flat-sequence {
          tunnel: w465 -> [w473]
          tunnel: w464 -> [w471]
          tunnel: [w472] -> w468
          tunnel: [w470] -> w467
          tunnel: [w469] -> w466
          tunnel: [w487] -> w462
          tunnel: w468 -> [w485]
          tunnel: w467 -> [w489]
          tunnel: w466 -> [_]
          tunnel: [w488] -> w461
          frame #0 {
            n181 = local read "Screen Index"() -> (w469:i32)
            n182 = case shown="0, Default" w469 {
              selector: w469 -> [_ w481]
              tunnel: w473 -> [w475 w477]
              tunnel: [w475 w479] -> w472
              tunnel: w471 -> [w474 w480]
              tunnel: [w474 w480] -> w470
              frame -1, 2 {
              }
              frame 0, Default {
                n183 = invoke on="Sub Panel" class="SubPnl" method="Remove VI"(error in=w477) -> (error out=w476:errorcluster)  [unwired: 2 in, 2 out]
                n184 = Index Array(array=w480, index=w481) -> (element=w478:refnum<vi>)
                n185 = call "if VI is running stop VI.vi"("error in (no error)"=w476, "VI in"=w478) -> ("error out"=w479:errorcluster)  [unwired: 8 in, 1 out]
              }
            }
          }
          frame #1 {
            n186 = Index Array(array=w489, index=4) -> (element=w483:refnum<vi>)
            n187 = property class="VI"(reference=w483, error in=w485) -> (error out=w484:errorcluster, "Exec.State"=w482:T5)  [unwired: 1 out]
            n188 = case shown="\"Idle\", Default" w482 {
              tunnel: w484 -> [w492 w497]
              tunnel: [w492 w494] -> w487
              tunnel: w489 -> [_ w498]
              tunnel: [7 w496] -> w488
              frame "Bad" {
                n189 = One Button Dialog(message="Manual Mode  is Running") -> ()  [unwired: 1 in, 1 out]
              }
              frame "Idle", Default {
                w496 = 2 ("index")
                n190 = local write "Screen Index"(w496) -> ()
                n191 = Index Array(array=w498, index=w496) -> (element=w499:refnum<vi>)
                n192 = call "if VI is idle run VI.vi"("error in (no error)"=w497, "VI in"=w499) -> ("error out"=w493:errorcluster, "VI out"=w495:refnum<vi>)  [unwired: 8 in]
                n193 = invoke on="Sub Panel" class="SubPnl" method="Insert VI"(error in=w493, "VI Ref"=w495) -> (error out=w494:errorcluster)  [unwired: 2 in, 3 out]
              }
            }
          }
        }
        n194 = call "Change menu button color as per screen index.vi"("error in (no error)"=w462, "Screen Index"=w461, "Array"=w463) -> ("error out"=w460:errorcluster)  [unwired: 8 in]
      }
      event "MANUAL": Value Change {
        n195 = event-data() -> ()  [unwired: 1 in, 1 out]
        n196 = invoke on="Sub Panel" class="SubPnl" method="Remove VI"(error in=w502) -> (error out=w506:errorcluster)  [unwired: 2 in, 2 out]
        n197 = flat-sequence {
          tunnel: w506 -> [w513]
          tunnel: w503 -> [w511]
          tunnel: [w512] -> w508
          tunnel: [w510] -> w507
          tunnel: [w530] -> w505
          tunnel: w508 -> [w522]
          tunnel: w507 -> [w528]
          tunnel: [w529] -> w504
          frame #0 {
            n198 = local read "Screen Index"() -> (w509:i32)
            n199 = case shown="-1, 2" w509 {
              selector: w509 -> [_ w520]
              tunnel: w513 -> [w515 w518]
              tunnel: [w515 w517] -> w512
              tunnel: w511 -> [w514 w519]
              tunnel: [w514 w519] -> w510
              frame -1, 2 {
              }
              frame 0, Default {
                n200 = Index Array(array=w519, index=w520) -> (element=w516:refnum<vi>)
                n201 = call "if VI is running stop VI.vi"("error in (no error)"=w518, "VI in"=w516) -> ("error out"=w517:errorcluster)  [unwired: 8 in, 1 out]
              }
            }
          }
          frame #1 {
            n202 = Index Array(array=w528, index=3) -> (element=w523:refnum<vi>)
            n203 = property class="VI"(reference=w523, error in=w522) -> (error out=w526:errorcluster, "Exec.State"=w525:T5)  [unwired: 1 out]
            n204 = case shown="\"Idle\", Default" w525 {
              tunnel: w526 -> [w531 w533]
              tunnel: [TRUE FALSE] -> w524
              tunnel: [w531 w533] -> w521
              frame "Idle", Default {
              }
              frame "Run top level", "Running" {
              }
            }
            n205 = case shown="True" w524 {
              tunnel: w528 -> [_ w544]
              tunnel: [w536 w543] -> w530
              tunnel: w521 -> [w536 w542]
              tunnel: [3 ("index") w538] -> w529
              frame False {
                n206 = One Button Dialog(message="Auto Cycle is Running Go to Auto Cycle and Press EXIT") -> ()  [unwired: 1 in, 1 out]
              }
              frame True {
                w538 = 4 ("index")
                n207 = Index Array(array=w544, index=w538) -> (element=w539:refnum<vi>)
                n208 = call "if VI is idle run VI.vi"("error in (no error)"=w542, "VI in"=w539) -> ("error out"=w541:errorcluster, "VI out"=w540:refnum<vi>)  [unwired: 8 in]
                n209 = local write "Screen Index"(w538) -> ()
                n210 = invoke on="Sub Panel" class="SubPnl" method="Insert VI"(error in=w541, "VI Ref"=w540) -> (error out=w543:errorcluster)  [unwired: 2 in, 3 out]
              }
            }
          }
        }
        n211 = call "Change menu button color as per screen index.vi"("error in (no error)"=w505, "Screen Index"=w504, "Array"=w501) -> ("error out"=w500:errorcluster)  [unwired: 8 in]
      }
      event "REPORT": Value Change {
        n212 = event-data() -> ()  [unwired: 1 in, 3 out]
        n213 = invoke on="Sub Panel" class="SubPnl" method="Remove VI"(error in=w545) -> (error out=w550:errorcluster)  [unwired: 2 in, 2 out]
        n214 = flat-sequence {
          tunnel: w550 -> [w559]
          tunnel: w553 -> [w556]
          tunnel: [w558] -> w552
          tunnel: [w555] -> w551
          tunnel: [w572] -> w548
          tunnel: w552 -> [w571]
          tunnel: w551 -> [w573]
          tunnel: [w567] -> w546
          frame #0 {
            n215 = local read "Screen Index"() -> (w557:i32)
            n216 = case shown="-1, 2" w557 {
              selector: w557 -> [_ w566]
              tunnel: w559 -> [w561 w564]
              tunnel: [w561 w563] -> w558
              tunnel: w556 -> [w560 w565]
              tunnel: [w560 w565] -> w555
              frame -1, 2 {
              }
              frame 0, Default {
                n217 = Index Array(array=w565, index=w566) -> (element=w562:refnum<vi>)
                n218 = call "if VI is running stop VI.vi"("error in (no error)"=w564, "VI in"=w562) -> ("error out"=w563:errorcluster)  [unwired: 8 in, 1 out]
              }
            }
          }
          frame #1 {
            w567 = 3 ("index")
            n219 = local write "Screen Index"(w567) -> ()
            n220 = Index Array(array=w573, index=w567) -> (element=w568:refnum<vi>)
            n221 = call "if VI is idle run VI.vi"("error in (no error)"=w571, "VI in"=w568) -> ("error out"=w570:errorcluster, "VI out"=w569:refnum<vi>)  [unwired: 8 in]
            n222 = invoke on="Sub Panel" class="SubPnl" method="Insert VI"(error in=w570, "VI Ref"=w569) -> (error out=w572:errorcluster)  [unwired: 2 in, 3 out]
          }
        }
        n223 = call "Change menu button color as per screen index.vi"("error in (no error)"=w548, "Screen Index"=w546, "Array"=w547) -> ("error out"=w549:errorcluster)  [unwired: 8 in]
      }
      event "andon": Value Change {
        n224 = event-data() -> ()  [unwired: 1 in, 3 out]
        n225 = invoke on="Sub Panel" class="SubPnl" method="Remove VI"(error in=w574) -> (error out=w579:errorcluster)  [unwired: 2 in, 2 out]
        n226 = flat-sequence {
          tunnel: w579 -> [w588]
          tunnel: w582 -> [w585]
          tunnel: [w587] -> w581
          tunnel: [w584] -> w580
          tunnel: [w601] -> w577
          tunnel: w581 -> [w600]
          tunnel: w580 -> [w602]
          tunnel: [w596] -> w576
          frame #0 {
            n227 = local read "Screen Index"() -> (w586:i32)
            n228 = case shown="-1, 2" w586 {
              selector: w586 -> [_ w595]
              tunnel: w588 -> [w590 w593]
              tunnel: [w590 w592] -> w587
              tunnel: w585 -> [w589 w594]
              tunnel: [w589 w594] -> w584
              frame -1, 2 {
              }
              frame 0, Default {
                n229 = Index Array(array=w594, index=w595) -> (element=w591:refnum<vi>)
                n230 = call "if VI is running stop VI.vi"("error in (no error)"=w593, "VI in"=w591) -> ("error out"=w592:errorcluster)  [unwired: 8 in, 1 out]
              }
            }
          }
          frame #1 {
            w596 = 6 ("index")
            n231 = local write "Screen Index"(w596) -> ()
            n232 = Index Array(array=w602, index=w596) -> (element=w597:refnum<vi>)
            n233 = call "if VI is idle run VI.vi"("error in (no error)"=w600, "VI in"=w597) -> ("error out"=w599:errorcluster, "VI out"=w598:refnum<vi>)  [unwired: 8 in]
            n234 = invoke on="Sub Panel" class="SubPnl" method="Insert VI"(error in=w599, "VI Ref"=w598) -> (error out=w601:errorcluster)  [unwired: 2 in, 3 out]
          }
        }
        n235 = call "Change menu button color as per screen index.vi"("error in (no error)"=w577, "Screen Index"=w576, "Array"=w575) -> ("error out"=w578:errorcluster)  [unwired: 8 in]
      }
      event "Hardware Setting": Value Change {
        n236 = event-data() -> ()  [unwired: 1 in, 3 out]
        n237 = invoke on="Sub Panel" class="SubPnl" method="Remove VI"(error in=w603) -> (error out=w608:errorcluster)  [unwired: 2 in, 2 out]
        n238 = flat-sequence {
          tunnel: w608 -> [w617]
          tunnel: w611 -> [w614]
          tunnel: [w616] -> w610
          tunnel: [w613] -> w609
          tunnel: [w630] -> w606
          tunnel: w610 -> [w629]
          tunnel: w609 -> [w631]
          tunnel: [w625] -> w605
          frame #0 {
            n239 = local read "Screen Index"() -> (w615:i32)
            n240 = case shown="-1, 2" w615 {
              selector: w615 -> [_ w624]
              tunnel: w617 -> [w619 w622]
              tunnel: [w619 w621] -> w616
              tunnel: w614 -> [w618 w623]
              tunnel: [w618 w623] -> w613
              frame -1, 2 {
              }
              frame 0, Default {
                n241 = Index Array(array=w623, index=w624) -> (element=w620:refnum<vi>)
                n242 = call "if VI is running stop VI.vi"("error in (no error)"=w622, "VI in"=w620) -> ("error out"=w621:errorcluster)  [unwired: 8 in, 1 out]
              }
            }
          }
          frame #1 {
            w625 = 4 ("index")
            n243 = local write "Screen Index"(w625) -> ()
            n244 = Index Array(array=w631, index=w625) -> (element=w626:refnum<vi>)
            n245 = call "if VI is idle run VI.vi"("error in (no error)"=w629, "VI in"=w626) -> ("error out"=w628:errorcluster, "VI out"=w627:refnum<vi>)  [unwired: 8 in]
            n246 = invoke on="Sub Panel" class="SubPnl" method="Insert VI"(error in=w628, "VI Ref"=w627) -> (error out=w630:errorcluster)  [unwired: 2 in, 3 out]
          }
        }
        n247 = call "Change menu button color as per screen index.vi"("error in (no error)"=w606, "Screen Index"=w605, "Array"=w604) -> ("error out"=w607:errorcluster)  [unwired: 8 in]
      }
      event "Shift Setting": Value Change {
        n248 = event-data() -> ()  [unwired: 1 in, 3 out]
        n249 = invoke on="Sub Panel" class="SubPnl" method="Remove VI"(error in=w632) -> (error out=w637:errorcluster)  [unwired: 2 in, 2 out]
        n250 = flat-sequence {
          tunnel: w637 -> [w646]
          tunnel: w640 -> [w643]
          tunnel: [w645] -> w639
          tunnel: [w642] -> w638
          tunnel: [w659] -> w633
          tunnel: w639 -> [w658]
          tunnel: w638 -> [w660]
          tunnel: [w654] -> w635
          frame #0 {
            n251 = local read "Screen Index"() -> (w644:i32)
            n252 = case shown="-1, 2" w644 {
              selector: w644 -> [_ w653]
              tunnel: w646 -> [w648 w651]
              tunnel: [w648 w650] -> w645
              tunnel: w643 -> [w647 w652]
              tunnel: [w647 w652] -> w642
              frame -1, 2 {
              }
              frame 0, Default {
                n253 = Index Array(array=w652, index=w653) -> (element=w649:refnum<vi>)
                n254 = call "if VI is running stop VI.vi"("error in (no error)"=w651, "VI in"=w649) -> ("error out"=w650:errorcluster)  [unwired: 8 in, 1 out]
              }
            }
          }
          frame #1 {
            w654 = 5 ("index")
            n255 = local write "Screen Index"(w654) -> ()
            n256 = Index Array(array=w660, index=w654) -> (element=w655:refnum<vi>)
            n257 = call "if VI is idle run VI.vi"("error in (no error)"=w658, "VI in"=w655) -> ("error out"=w657:errorcluster, "VI out"=w656:refnum<vi>)  [unwired: 8 in]
            n258 = invoke on="Sub Panel" class="SubPnl" method="Insert VI"(error in=w657, "VI Ref"=w656) -> (error out=w659:errorcluster)  [unwired: 2 in, 3 out]
          }
        }
        n259 = call "Change menu button color as per screen index.vi"("error in (no error)"=w633, "Screen Index"=w635, "Array"=w634) -> ("error out"=w636:errorcluster)  [unwired: 8 in]
      }
      event "Test Print": Value Change {
        n260 = event-data() -> ()  [unwired: 1 in, 3 out]
        n261 = invoke on="Sub Panel" class="SubPnl" method="Remove VI"(error in=w661) -> (error out=w666:errorcluster)  [unwired: 2 in, 2 out]
        n262 = flat-sequence {
          tunnel: w666 -> [w675]
          tunnel: w669 -> [w672]
          tunnel: [w674] -> w668
          tunnel: [w671] -> w667
          tunnel: [w688] -> w664
          tunnel: w668 -> [w687]
          tunnel: w667 -> [w689]
          tunnel: [w683] -> w663
          frame #0 {
            n263 = local read "Screen Index"() -> (w673:i32)
            n264 = case shown="-1, 2" w673 {
              selector: w673 -> [_ w682]
              tunnel: w675 -> [w677 w680]
              tunnel: [w677 w679] -> w674
              tunnel: w672 -> [w676 w681]
              tunnel: [w676 w681] -> w671
              frame -1, 2 {
              }
              frame 0, Default {
                n265 = Index Array(array=w681, index=w682) -> (element=w678:refnum<vi>)
                n266 = call "if VI is running stop VI.vi"("error in (no error)"=w680, "VI in"=w678) -> ("error out"=w679:errorcluster)  [unwired: 8 in, 1 out]
              }
            }
          }
          frame #1 {
            w683 = 9 ("index")
            n267 = local write "Screen Index"(w683) -> ()
            n268 = Index Array(array=w689, index=w683) -> (element=w684:refnum<vi>)
            n269 = call "if VI is idle run VI.vi"("error in (no error)"=w687, "VI in"=w684) -> ("error out"=w686:errorcluster, "VI out"=w685:refnum<vi>)  [unwired: 8 in]
            n270 = invoke on="Sub Panel" class="SubPnl" method="Insert VI"(error in=w686, "VI Ref"=w685) -> (error out=w688:errorcluster)  [unwired: 2 in, 3 out]
          }
        }
        n271 = call "Change menu button color as per screen index.vi"("error in (no error)"=w664, "Screen Index"=w663, "Array"=w662) -> ("error out"=w665:errorcluster)  [unwired: 8 in]
      }
      event "Home": Value Change {
        n272 = event-data() -> ()  [unwired: 1 in, 3 out]
        n273 = invoke on="Sub Panel" class="SubPnl" method="Remove VI"(error in=w690) -> (error out=w693:errorcluster)  [unwired: 2 in, 2 out]
        n274 = call "Change menu button color as per screen index.vi"("error in (no error)"=w693, "Screen Index"=-1, "Array"=w691) -> ("error out"=w692:errorcluster)  [unwired: 8 in]
      }
      event "EXIT": Value Change {
        n275 = event-data() -> ()  [unwired: 1 in, 1 out]
        n276 = Index Array(array=w698, index=2) -> (element=w704:refnum<vi>)
        n277 = Build Array(w704) -> (w703:refnum<vi>[])
        n278 = for {
          tunnel: w698 -> [w727]
          tunnel: [w726] -> w706 mode=indexing
          shift-right: [w725] -> w700
          shift-left: w705 -> [w724]
          tunnel: w703 -> [w723] mode=indexing
          n279 = property class="VI"(reference=w723, error in=w724) -> (error out=w729:errorcluster, "Exec.State"=w728:T5)  [unwired: 1 out]
          n280 = case shown="\"Run top level\", \"Running\"" w728 {
            tunnel: w729 -> [w730 w732]
            tunnel: w727 -> [_ _]
            tunnel: [TRUE FALSE] -> w726
            tunnel: [w730 w732] -> w725
            frame "Idle", Default {
            }
            frame "Run top level", "Running" {
            }
          }
        }
        n281 = And Array Elements(Boolean array=w706) -> (logical AND=w702:bool)
        n282 = case shown="False" w702 {
          tunnel: [FALSE TRUE] -> w697
          tunnel: w700 -> [w711 w715]
          tunnel: [w711 w714] -> w699
          tunnel: w698 -> [_ w713]
          frame False {
            n283 = One Button Dialog(message="Auto Cycle  is Running") -> ()  [unwired: 1 in, 1 out]
          }
          frame True {
            n284 = invoke on="Sub Panel" class="SubPnl" method="Remove VI"(error in=w715) -> (error out=w716:errorcluster)  [unwired: 2 in, 2 out]
            n285 = for {
              shift-right: [w722] -> w714
              shift-left: w716 -> [w721]
              tunnel: w713 -> [w717] mode=indexing
              n286 = call "if VI is running stop VI.vi"("error in (no error)"=w721, "VI in"=w717) -> ("error out"=w720:errorcluster, "VI out"=w719:refnum<vi>)  [unwired: 8 in]
              n287 = call <vilib>:"Clear Errors.vi"("error in (no error)"=w720) -> ("error out"=w718:errorcluster)  [unwired: 5 in, 1 out]
              n288 = Close Reference(reference=w719, error in (no error)=w718) -> (error out=w722:errorcluster)
            }
          }
        }
        n289 = call "Change menu button color as per screen index.vi"("error in (no error)"=w699, "Screen Index"=-1, "Array"=w701) -> ("error out"=w696:errorcluster)  [unwired: 8 in]
      }
      event "Remove": Value Change {
        n290 = event-data() -> ()  [unwired: 1 in, 1 out]
        n291 = invoke on="Sub Panel" class="SubPnl" method="Remove VI"(error in=w734) -> (error out=w736:errorcluster)  [unwired: 2 in, 2 out]
        n292 = call "Change menu button color as per screen index.vi"("error in (no error)"=w736, "Screen Index"=-1, "Array"=w735) -> ("error out"=w737:errorcluster)  [unwired: 8 in]
      }
      event Timeout {
        n293 = event-data() -> ()  [unwired: 1 in, 1 out]
        n294 = global read "Global 1.vi" "BARCODE RECIPE"() -> (w749:string)
        n295 = global read "Global 1.vi" "MODEL SELECTION"() -> (w750:bool)
        n296 = global read "Login Details.vi" "User Name"() -> (→"user name":string)
        n297 = Format Date/Time String(time format string (%c)="%d/ %m/ %Y\n%H:%M:%S") -> (date/time string=→"datetime":string)  [unwired: 2 in]
        n298 = Empty String/Path?(string/path=w749) -> (empty?=w748:bool)
        n299 = Or(x="Check 2", y=w750) -> (x .or. y?=w754:bool)
        n300 = global read "Global 1.vi" "REMOVE VI"() -> (w751:bool)
        n301 = case shown="True" w754 {
          tunnel: w752 -> [w782 w787]
          tunnel: [w782 w786] -> w741
          tunnel: w748 -> [_ w784]
          frame False {
          }
          frame True {
            n302 = flat-sequence {
              tunnel: w787 -> [w791]
              tunnel: [w789] -> w785
              tunnel: w784 -> [w788]
              tunnel: [w788] -> w783
              tunnel: [w794] -> w786
              tunnel: w785 -> [w795]
              tunnel: w783 -> [w793]
              frame #0 {
                n303 = invoke on="Sub Panel" class="SubPnl" method="Remove VI"(error in=w791) -> (error out=w789:errorcluster)  [unwired: 2 in, 2 out]
                n304 = global write "Global 1.vi" "MODEL SELECTION"(FALSE ("remove_VI")) -> ()
                n305 = local write "Check 2"(FALSE ("Check")) -> ()
              }
              frame #1 {
                n306 = case shown="False" w793 {
                  tunnel: w795 -> [w797 w799]
                  tunnel: [w796 w799] -> w794
                  frame False {
                    n307 = property on="auto" class="Bool (strict)"(error in=w797, "Val(Sgnl)"=TRUE ("Value (Signaling)")) -> (error out=w796:errorcluster)  [unwired: 1 in, 1 out]
                  }
                  frame True {
                  }
                }
              }
            }
          }
        }
        n308 = Or(x="Check", y=w751) -> (x .or. y?=w779:bool)
        n309 = case shown="False" w779 {
          selector: w779 -> [_ w814]
          frame False {
          }
          frame True {
            n310 = global write "Global 1.vi" "REMOVE VI"(FALSE ("remove_VI")) -> ()
            n311 = property on="Remove" class="Bool (strict)"("Val(Sgnl)"=w814) -> ()  [unwired: 2 in, 2 out]
            n312 = local write "Check"(FALSE ("Check")) -> ()
          }
        }
        n313 = global read "Login Details.vi" "Authority"() -> (w775:T2)
        n314 = Unbundle By Name(w775) -> ("SCREEN 2"=w773:bool, "SCREEN 3"=w772:bool, "SCREEN 4"=w771:bool, "SCREEN 5"=w770:bool, "SCREEN 6"=w769:bool, "SCREEN 7"=w768:bool, "SCREEN 8"=w767:bool, "SCREEN 9"=w766:bool, "SCREEN 10"=w765:bool, "SCREEN 11"=w764:bool, "SCREEN 12"=w763:bool, "SCREEN 13"=w762:bool, "SCREEN 14"=w761:bool, "SCREEN 15"=w760:bool, "SCREEN 16"=w759:bool, "SCREEN 17"=w758:bool, "SCREEN 18"=w757:bool, "SCREEN 19"=w756:bool, "SCREEN 20"=w755:bool)  [unwired: 1 out]
        n315 = control-ref of="Hardware Setting"() -> (w744:refnum<vi>)
        n316 = control-ref of="Shift Setting"() -> (w743:refnum<vi>)
        n317 = control-ref of="REPORT"() -> (w745:refnum<vi>)
        n318 = control-ref of="USER MANGMENT"() -> (w747:refnum<vi>)
        n319 = control-ref of="AUTO MODE"() -> (w746:refnum<vi>)
        n320 = Build Array(w747, w746, w745, w744, w743) -> (w742:refnum<vi>[])
        n321 = Build Array(w773, w772, w771, w770, w769, w768, w767, w766, w765, w764, w763, w762, w761, w760, w759, w758, w757, w756, w755) -> (w774:bool[])
        n322 = for {
          tunnel: w774 -> [w802] mode=indexing
          tunnel: w742 -> [w803] mode=indexing
          tunnel: w741 -> [w801]
          tunnel: [w800] -> w740
          n323 = case shown="True" w802 {
            tunnel: w803 -> [w806 w810]
            tunnel: w801 -> [w805 w809]
            tunnel: [w804 w808] -> w800
            frame True {
              n324 = property class="Bool"(reference=w806, error in=w805, "DisabledEnum"=T3."Enabled" ("Disabled")) -> (error out=w804:errorcluster)  [unwired: 1 out]
            }
            frame False {
              n325 = property class="Bool"(reference=w810, error in=w809, "DisabledEnum"=T3."Disabled and Grayed Out" ("Disabled")) -> (error out=w808:errorcluster)  [unwired: 1 out]
            }
          }
        }
      }
    }
  }
  n326 = call <vilib>:"Clear Errors.vi"("error in (no error)"=w22) -> ("error out"=w12:errorcluster)  [unwired: 5 in, 1 out]
  n327 = disable-structure shown="Disabled" {
    disable-tunnel: w1 -> [w815 _]
    frame Disabled {
      n328 = Quit LabVIEW(quit? (T)=w815) -> ()
    }
    frame Enabled {
    }
  }
  n329 = call "PADMINI_STOP_ALL.vi"("Enum"=enum16{"Read", "Write"}."Write", "error in (no error)"=w12, "Boolean"=TRUE) -> ("error out"=w9:errorcluster)  [unwired: 7 in, 1 out]
  n330 = call <vilib>:"Clear Errors.vi"("error in (no error)"=w9) -> ("error out"=w35:errorcluster)  [unwired: 5 in, 1 out]
  n331 = property class="App"(error in=w35) -> (error out=w36:errorcluster, "App.Kind"=w37:T6)  [unwired: 1 in, 1 out]
  n332 = case shown="\"Run Time System\"" w37 {
    tunnel: w36 -> [w816 w818]
    tunnel: [w816 w817] -> w34
    frame Default {
    }
    frame "Run Time System" {
      n333 = invoke class="VI" method="FP.Close"(error in=w818) -> (error out=w817:errorcluster)  [unwired: 2 in, 2 out]
    }
  }
  "error out 2" <- w34
